vi "Wait and Convert Notification.vi"   [LabVIEW 2024]
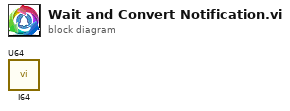
[diagram p0: block diagram]
diagram:
  n1 = call "I64.vi"() -> ()  [unwired: 8 in, 4 out]
  n2 = call "U64.vi"() -> ()  [unwired: 8 in, 4 out]
